vi "Get Child Coordinates.vi"(8 "error in (no error)":errorcluster, 10 "Child hWnd":u32, 11 "Parent hWnd":u32) -> (0 "error out":errorcluster, 2 "Absolute":T1, 3 "Relative":T1)   [LabVIEW 2011]
uses:
  Windows Utilities/Controls/Window Rectangle (hwnd).ctl
  user32.dll
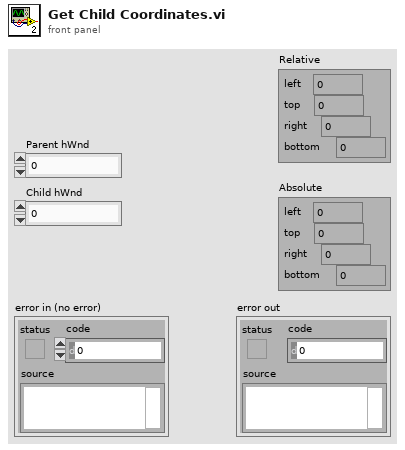
[diagram p1: front panel]
types:
  T1 = typedef "Window Rectangle (hwnd).ctl" = cluster{"left":i16, "top":i16, "right":i16, "bottom":i16}
  T2 = cluster{"LPPoints[0]":i32, "LPPoints[1]":i32, "LPPoints[2]":i32, "LPPoints[3]":i32}
  T3 = cluster{"RECT[0]":i32, "RECT[1]":i32, "RECT[2]":i32, "RECT[3]":i32}
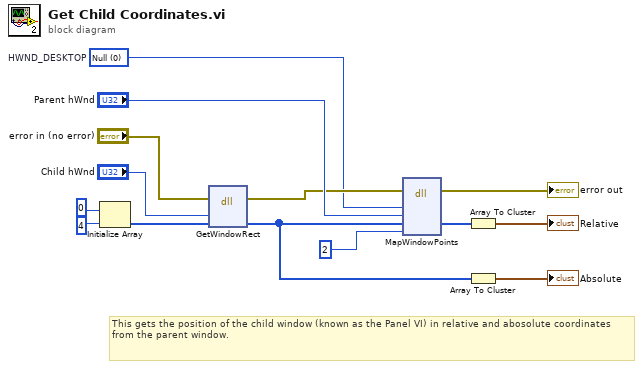
[diagram p0: block diagram]
diagram:
  w3 = u32 0 items=["Null"]  # HWND_DESKTOP
  # "This gets the position of the child window (known as the Panel VI) in relative and abosolute coordinates from the parent window."
  n1 = Initialize Array(0, 4) -> (w12:i32[])
  n2 = dll-call lib="USER32.DLL" fn="GetWindowRect"(error in="error in (no error)", "hWnd"="Child hWnd", "RECT"=w12) -> (error out=w4:errorcluster, "RECT"=w7:i32[])  [unwired: 3 in, 2 out]
  n3 = dll-call lib="USER32.DLL" fn="MapWindowPoints"(error in=w4, "hWndFrom"=w3, "hWndTo"="Parent hWnd", "LPPoints"=w7, "cPoints"=u32 2) -> (error out=→"error out":errorcluster, "LPPoints"=w10:i32[])  [unwired: 4 in, 3 out]
  n4 = Array To Cluster(array=w10) -> (cluster=→"Relative":T2)
  n5 = Array To Cluster(array=w7) -> (cluster=→"Absolute":T3)
